vi "Run Script File.vi"(8 "error in (no error)":errorcluster, 11 "pattern":string) -> (0 "error out":errorcluster)   [LabVIEW 2020]
uses:
  <userlib>/_NEVSTOP/Communicable State Machine(CSM)/Communicable State Machine.lvlib
  <userlib>/_NEVSTOP/Communicable State Machine(CSM)/_tool/_file/csm-file-support.lvlib
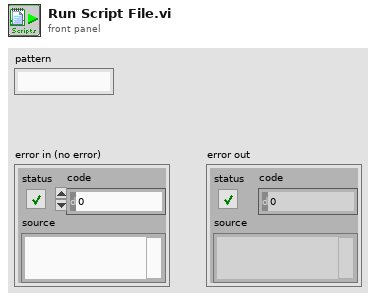
[diagram p1: front panel]
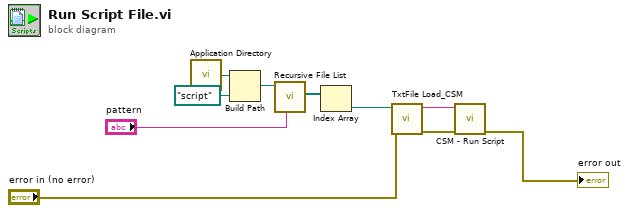
[diagram p0: block diagram]
diagram:
  n1 = call <vilib>:"Application Directory.vi"() -> ("Application Directory"=w1:path)
  n2 = Build Path(base path=w1, name or relative path=path "script") -> (appended path=w3:path)
  n3 = call <vilib>:"Recursive File List.vi"("pattern"="pattern", "Folder Path"=w3) -> ("All Files in Dir"=w4:path[])  [unwired: 5 in, 4 out]
  n4 = Index Array(array=w4) -> (element=w5:path)  [unwired: 1 in]
  n5 = call <userlib>:"TxtFile Load_CSM.vi"("error in (no error)"="error in (no error)", "Path"=w5) -> ("error out"=w8:errorcluster, "Text"=w7:string)  [unwired: 8 in]
  n6 = call <userlib>:"CSM - Run Script.vi"("CSM Scripts"=w7, "error in (no error)"=w8) -> ("error out"=→"error out":errorcluster)  [unwired: 11 in, 2 out]
